vi "BRig_RT_panel_cue_v1,17.vi"(7 "input_setValues":bool, 11 "input_dataExp":u16[](array[numeric])) -> (3 "output_dataExp":u16[](array[numeric]))   [LabVIEW 2014]
panel:
  in  "Cue1B_LorR":bool
  in  "Cue1B_Prob":u16
  in  "sp__Cue1B":u16(slide)=2 max=2 step=1 scale=0.0..2.0
  in  "Audio_Amp__Cue1B":u16=100 caption="Amp"
  in  "Audio_Freq__Cue1B":u16=5 caption="Freq [kHz]" max=14 step=1
  in  "Cue1BSwitch_Prob":u16
  in  "Cue1BSwitch":u16(slide) max=3 step=1 scale=0.0..3.0
  in  "Cue2Switch_Count_PostR":u16
  in  "Cue2Switch_Prob_PostR":u16
  in  "Cue2Switch_PostR":u16(slide) max=3 step=1 scale=0.0..3.0
  in  "Cue2Switch_Count_PreR":u16
  in  "Cue2Switch_Count_First":u16
  in  "Cue2Switch_Prob_PreR":u16
  in  "Cue2Switch_PreR":u16(slide) max=3 step=1 scale=0.0..3.0
  in  "Cue2Switch_Prob_First":u16
  in  "Cue2Switch_First":u16(slide) max=3 step=1 scale=0.0..3.0
  in  "CueLed_baseline":bool
  in  "CueSwitch_Count_PostR":u16
  in  "CueSwitch_Prob_PostR":u16
  in  "CueSwitch_PostR":u16(slide) max=3 step=1 scale=0.0..3.0
  in  "CueSwitch_Count_PreR":u16
  in  "CueSwitch_Count_First":u16
  in  "CueSwitch_Prob_PreR":u16
  in  "CueSwitch_PreR":u16(slide) max=3 step=1 scale=0.0..3.0
  in  "CueSwitch_Prob_First":u16
  in  "CueSwitch_First":u16(slide) max=3 step=1 scale=0.0..3.0
  in  "CueLed_Freq":u16=10
  in  "CueLed_Tpeak":u16=2
  in  "sp_RightSpout":u16(slide)=2 max=2 step=1 scale=0.0..2.0
  in  "sp_LeftSpout":u16(slide)=2 max=2 step=1 scale=0.0..2.0
  in  "Audio_Amp__R":u16=100 caption="Amp"
  in  "Audio_Freq__R":u16=5 caption="Freq [kHz]" max=14 step=1
  in  "Audio_Amp__L":u16=100 caption="Amp"
  in  "Audio_Freq__L":u16=5 caption="Freq [kHz]" max=14 step=1
  # "Cue State\n                                             Cue Type         LED Probability    Count"
  # "Cue LED Parameters"
  # "Audio or LED"
  # "Frequency\n[Hz]"
  # "1A     1B"
  # "Timing [ms]\n                    Peak Width"
  # "1A\n1B"
  # "First"
  # "Pre Reward"
  # "Audio Parameters"
  # "Post Reward"
  # "Left                  Right"
  # "Frequency\n[kHz]"
  # "Cue2 State\n                                             Cue Type     LED Probability    Count"
  # "1A\n1B"
  # "2"
  # "Audio or LED"
  # "First"
  # "Amp\n(0 - 32,000)"
  # "1A\n1B"
  # "2"
  # "Pre Reward"
  # "1A  1B"
  # "2"
  # "Speaker\nPattern\nDuring Cue"
  # "Post Reward"
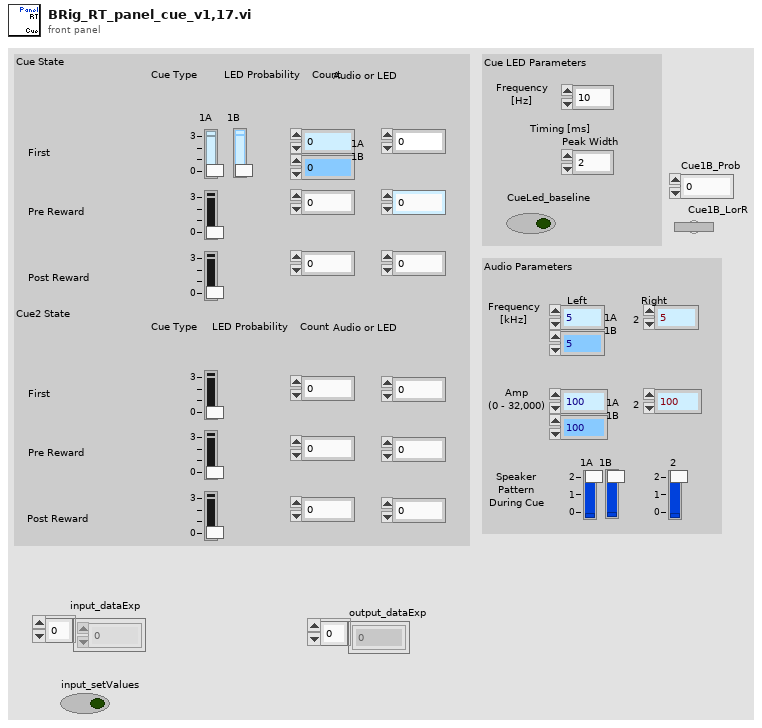
[diagram p1: front panel]
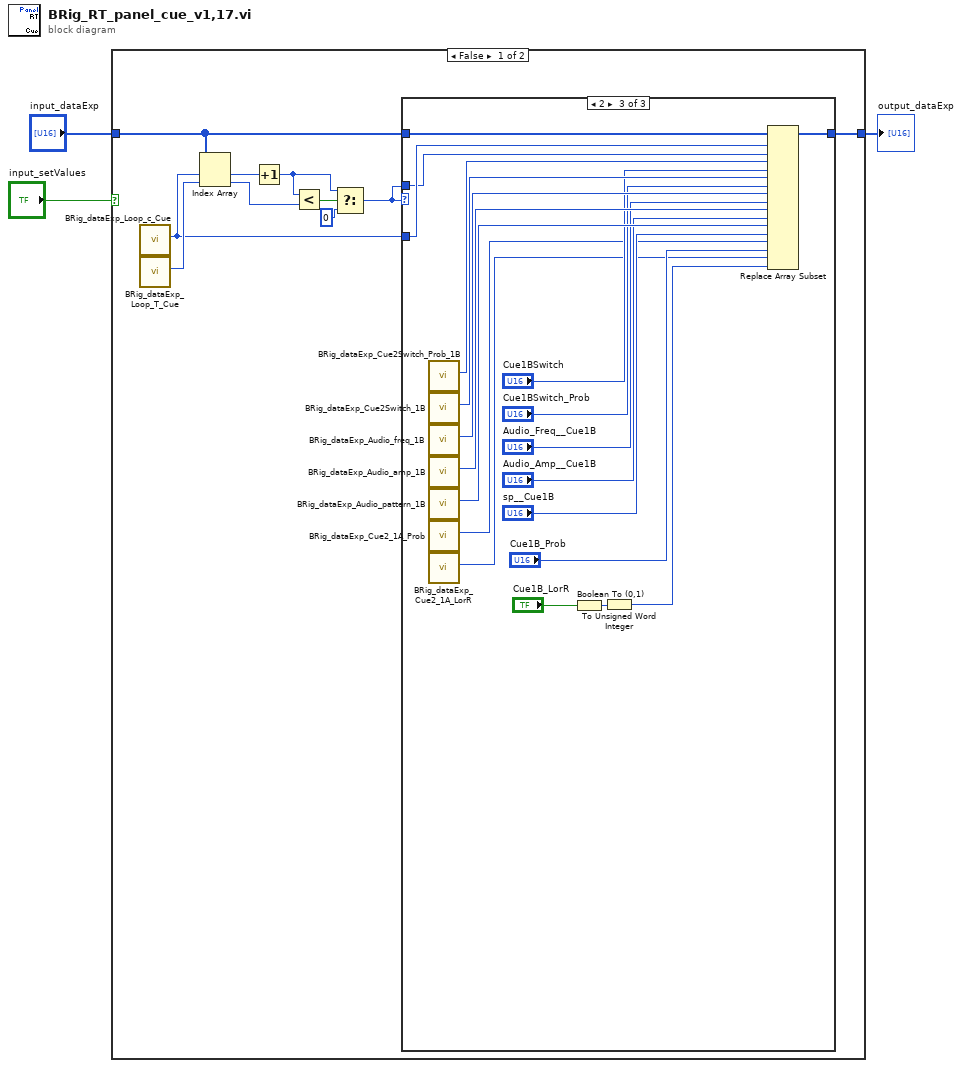
[diagram p0: block diagram]
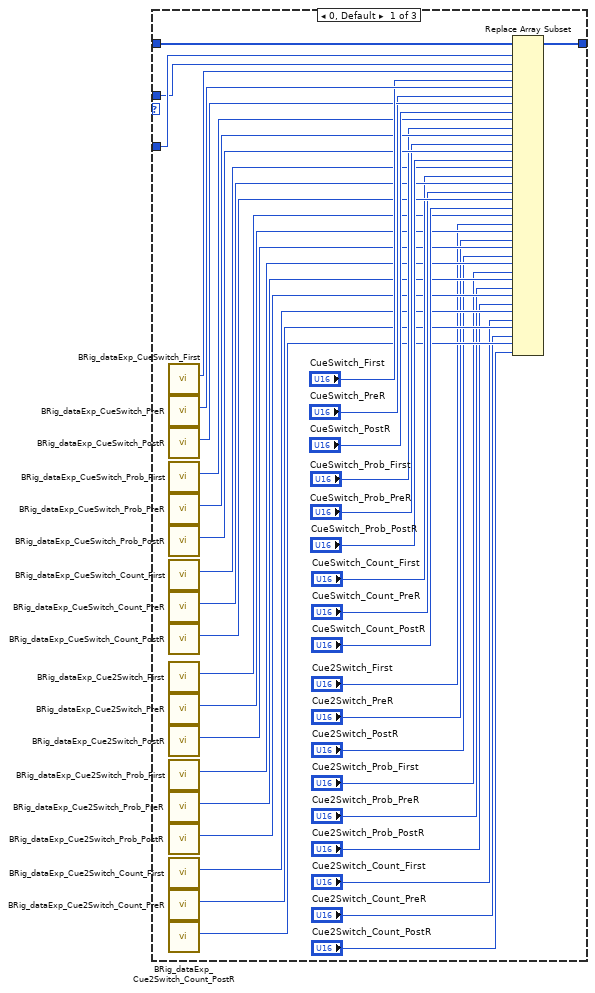
[diagram p2: hidden frame]
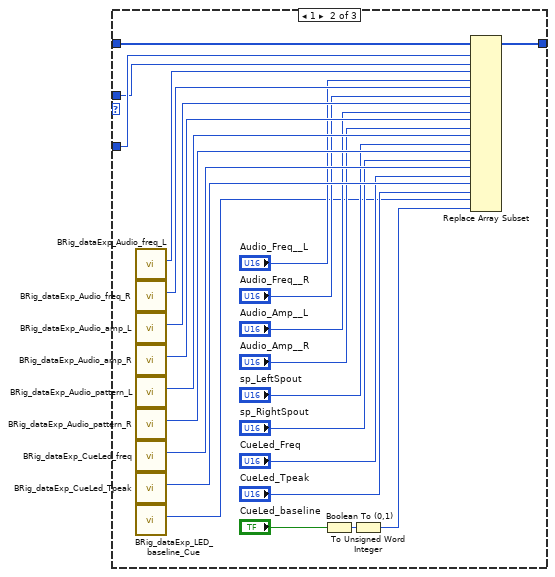
[diagram p3: hidden frame]
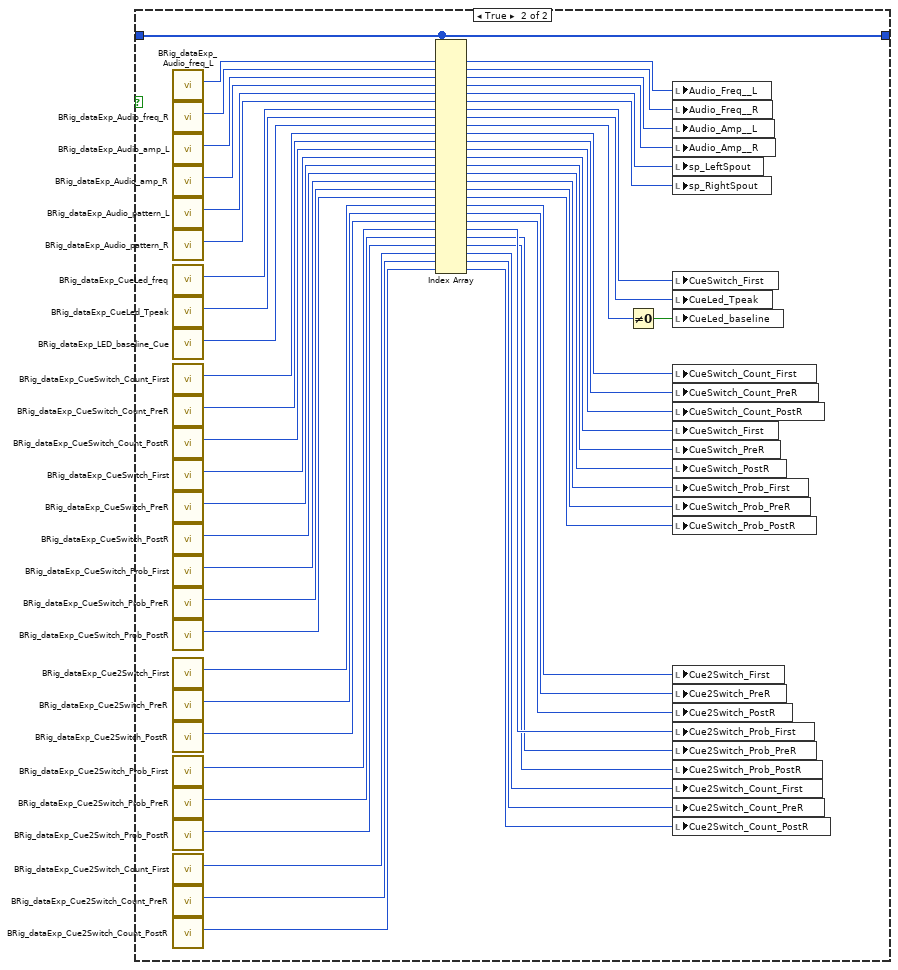
[diagram p4: hidden frame]
diagram:
  n1 = case shown="False" "input_setValues" {
    tunnel: "input_dataExp" -> [w7 w153]
    tunnel: [w6 w153] -> w2
    frame False {
      n2 = call "BRig_dataExp_Loop_c_Cue.vi"() -> ("output_Loop_c_Cue"=w5:i32)  [unwired: 11 in]
      n3 = call "BRig_dataExp_Loop_T_Cue.vi"() -> ("output_Loop_T_Cue"=w13:i32)  [unwired: 11 in]
      n4 = Index Array(array=w7, index #1=w5, index #2=w13) -> (element #1=w12:u16, element #2=w11:u16)
      n5 = Increment(x=w12) -> (x+1=w9:u16)
      n6 = Less?(x=w9, y=w11) -> (x < y?=w10:bool)
      n7 = Select(t=w9, s=w10, f=u16 0) -> (s? t:f=w4:u16)
      n8 = case shown="2" w4 {
        tunnel: w7 -> [w53 w77 w97]
        tunnel: [w34 w76 w96] -> w6
        tunnel: w5 -> [w33 w75 w95]
        tunnel: w4 -> [w32 w74 w94]
        frame 0, Default {
          n9 = call "BRig_dataExp_CueSwitch_First.vi"() -> ("output_CueSwitch_First"=w52:i32)  [unwired: 11 in]
          n10 = call "BRig_dataExp_CueSwitch_PreR.vi"() -> ("output_CueSwitch_PreR"=w51:i32)  [unwired: 11 in]
          n11 = call "BRig_dataExp_CueSwitch_PostR.vi"() -> ("output_CueSwitch_PostR"=w49:i32)  [unwired: 11 in]
          n12 = call "BRig_dataExp_CueSwitch_Prob_First.vi"() -> ("output_CueSwitch_Prob_First"=w46:i32)  [unwired: 11 in]
          n13 = call "BRig_dataExp_CueSwitch_Prob_PreR.vi"() -> ("output_CueSwitch_Prob_PreR"=w45:i32)  [unwired: 11 in]
          n14 = call "BRig_dataExp_CueSwitch_Prob_PostR.vi"() -> ("output_CueSwitch_Prob_PostR"=w44:i32)  [unwired: 11 in]
          n15 = call "BRig_dataExp_CueSwitch_Count_First.vi"() -> ("output_CueSwitch_Count_First"=w40:i32)  [unwired: 11 in]
          n16 = call "BRig_dataExp_CueSwitch_Count_PreR.vi"() -> ("output_CueSwitch_Count_PreR"=w39:i32)  [unwired: 11 in]
          n17 = call "BRig_dataExp_CueSwitch_Count_PostR.vi"() -> ("output_CueSwitch_Count_PostR"=w38:i32)  [unwired: 11 in]
          n18 = call "BRig_dataExp_Cue2Switch_First.vi"() -> ("output_Cue2Switch_First"=w31:i32)  [unwired: 11 in]
          n19 = call "BRig_dataExp_Cue2Switch_PreR.vi"() -> ("output_Cue2Switch_PreR"=w30:i32)  [unwired: 11 in]
          n20 = call "BRig_dataExp_Cue2Switch_PostR.vi"() -> ("output_Cue2Switch_PostR"=w29:i32)  [unwired: 11 in]
          n21 = call "BRig_dataExp_Cue2Switch_Prob_First.vi"() -> ("output_Cue2Switch_Prob_First"=w28:i32)  [unwired: 11 in]
          n22 = call "BRig_dataExp_Cue2Switch_Prob_PreR.vi"() -> ("output_Cue2Switch_Prob_PreR"=w27:i32)  [unwired: 11 in]
          n23 = call "BRig_dataExp_Cue2Switch_Prob_PostR.vi"() -> ("output_Cue2Switch_Prob_PostR"=w26:i32)  [unwired: 11 in]
          n24 = call "BRig_dataExp_Cue2Switch_Count_First.vi"() -> ("output_Cue2Switch_Count_First"=w25:i32)  [unwired: 11 in]
          n25 = call "BRig_dataExp_Cue2Switch_Count_PreR.vi"() -> ("output_Cue2Switch_Count_PreR"=w24:i32)  [unwired: 11 in]
          n26 = call "BRig_dataExp_Cue2Switch_Count_PostR.vi"() -> ("output_Cue2Switch_Count_PostR"=w23:i32)  [unwired: 11 in]
          n27 = Replace Array Subset(array=w53, new element #1=w32, index #1=w33, new element #2="CueSwitch_First", index #2=w52, new element #3="CueSwitch_PreR", index #3=w51, new element #4="CueSwitch_PostR", index #4=w49, new element #5="CueSwitch_Prob_First", index #5=w46, new element #6="CueSwitch_Prob_PreR", index #6=w45, new element #7="CueSwitch_Prob_PostR", index #7=w44, new element #8="CueSwitch_Count_First", index #8=w40, new element #9="CueSwitch_Count_PreR", index #9=w39, new element #10="CueSwitch_Count_PostR", index #10=w38, new element #11="Cue2Switch_First", index #11=w31, new element #12="Cue2Switch_PreR", index #12=w30, new element #13="Cue2Switch_PostR", index #13=w29, new element #14="Cue2Switch_Prob_First", index #14=w28, new element #15="Cue2Switch_Prob_PreR", index #15=w27, new element #16="Cue2Switch_Prob_PostR", index #16=w26, new element #17="Cue2Switch_Count_First", index #17=w25, new element #18="Cue2Switch_Count_PreR", index #18=w24, new element #19="Cue2Switch_Count_PostR", index #19=w23) -> (w34:u16[])
        }
        frame 1 {
          n28 = call "BRig_dataExp_Audio_freq_L.vi"() -> ("output_Audio_freq__L"=w73:i32)  [unwired: 11 in]
          n29 = call "BRig_dataExp_Audio_freq_R.vi"() -> ("output_Audio_freq__R"=w72:i32)  [unwired: 11 in]
          n30 = call "BRig_dataExp_Audio_amp_L.vi"() -> ("output_Audio_amp__L"=w71:i32)  [unwired: 11 in]
          n31 = call "BRig_dataExp_Audio_amp_R.vi"() -> ("output_Audio_amp__R"=w70:i32)  [unwired: 11 in]
          n32 = call "BRig_dataExp_Audio_pattern_L.vi"() -> ("output_Audio_sp__L"=w69:i32)  [unwired: 11 in]
          n33 = call "BRig_dataExp_Audio_pattern_R.vi"() -> ("output_Audio_sp__R"=w68:i32)  [unwired: 11 in]
          n34 = call "BRig_dataExp_CueLed_freq.vi"() -> ("output_CueLed_Freq"=w67:i32)  [unwired: 11 in]
          n35 = call "BRig_dataExp_CueLed_Tpeak.vi"() -> ("output_CueLed_Tpeak"=w66:i32)  [unwired: 11 in]
          n36 = call "BRig_dataExp_LED_baseline_Cue.vi"() -> ("output_LED_baseline_Cue"=w57:i32)  [unwired: 11 in]
          n37 = Boolean To (0,1)(Boolean="CueLed_baseline") -> (0, 1=w55:i16)
          n38 = To Unsigned Word Integer(number=w55) -> (unsigned 16bit integer=w54:u16)
          n39 = Replace Array Subset(array=w77, new element #1=w74, index #1=w75, new element #2="Audio_Freq__L", index #2=w73, new element #3="Audio_Freq__R", index #3=w72, new element #4="Audio_Amp__L", index #4=w71, new element #5="Audio_Amp__R", index #5=w70, new element #6="sp_LeftSpout", index #6=w69, new element #7="sp_RightSpout", index #7=w68, new element #8="CueLed_Freq", index #8=w67, new element #9="CueLed_Tpeak", index #9=w66, new element #10=w54, index #10=w57) -> (w76:u16[])
        }
        frame 2 {
          n40 = call "BRig_dataExp_Cue2Switch_Prob_1B.vi"() -> ("output_Cue2Switch_Prob_1B"=w93:i32)  [unwired: 11 in]
          n41 = call "BRig_dataExp_Cue2Switch_1B.vi"() -> ("output_Cue2Switch_1B"=w92:i32)  [unwired: 11 in]
          n42 = call "BRig_dataExp_Audio_freq_1B.vi"() -> ("output_Audio_freq__1B"=w91:i32)  [unwired: 11 in]
          n43 = call "BRig_dataExp_Audio_amp_1B.vi"() -> ("output_Audio_amp__1B"=w90:i32)  [unwired: 11 in]
          n44 = call "BRig_dataExp_Audio_pattern_1B.vi"() -> ("output_Audio_sp__1B"=w89:i32)  [unwired: 11 in]
          n45 = call "BRig_dataExp_Cue2_1A_Prob.vi"() -> ("output_Cue2_1A_Prob"=w83:i32)  [unwired: 11 in]
          n46 = call "BRig_dataExp_Cue2_1A_LorR.vi"() -> ("output_Cue2_1A_LorR"=w81:i32)  [unwired: 11 in]
          n47 = Boolean To (0,1)(Boolean="Cue1B_LorR") -> (0, 1=w79:i16)
          n48 = To Unsigned Word Integer(number=w79) -> (unsigned 16bit integer=w78:u16)
          n49 = Replace Array Subset(array=w97, new element #1=w94, index #1=w95, new element #2="Cue1BSwitch", index #2=w93, new element #3="Cue1BSwitch_Prob", index #3=w92, new element #4="Audio_Freq__Cue1B", index #4=w91, new element #5="Audio_Amp__Cue1B", index #5=w90, new element #6="sp__Cue1B", index #6=w89, new element #7="Cue1B_Prob", index #7=w83, new element #8=w78, index #8=w81) -> (w96:u16[])
        }
      }
    }
    frame True {
      n50 = call "BRig_dataExp_Audio_freq_L.vi"() -> ("output_Audio_freq__L"=w152:i32)  [unwired: 11 in]
      n51 = call "BRig_dataExp_Audio_freq_R.vi"() -> ("output_Audio_freq__R"=w150:i32)  [unwired: 11 in]
      n52 = call "BRig_dataExp_Audio_amp_L.vi"() -> ("output_Audio_amp__L"=w148:i32)  [unwired: 11 in]
      n53 = call "BRig_dataExp_Audio_amp_R.vi"() -> ("output_Audio_amp__R"=w146:i32)  [unwired: 11 in]
      n54 = call "BRig_dataExp_Audio_pattern_L.vi"() -> ("output_Audio_sp__L"=w144:i32)  [unwired: 11 in]
      n55 = call "BRig_dataExp_Audio_pattern_R.vi"() -> ("output_Audio_sp__R"=w143:i32)  [unwired: 11 in]
      n56 = call "BRig_dataExp_CueLed_freq.vi"() -> ("output_CueLed_Freq"=w140:i32)  [unwired: 11 in]
      n57 = call "BRig_dataExp_CueLed_Tpeak.vi"() -> ("output_CueLed_Tpeak"=w138:i32)  [unwired: 11 in]
      n58 = call "BRig_dataExp_LED_baseline_Cue.vi"() -> ("output_LED_baseline_Cue"=w136:i32)  [unwired: 11 in]
      n59 = call "BRig_dataExp_CueSwitch_Count_First.vi"() -> ("output_CueSwitch_Count_First"=w133:i32)  [unwired: 11 in]
      n60 = call "BRig_dataExp_CueSwitch_Count_PreR.vi"() -> ("output_CueSwitch_Count_PreR"=w132:i32)  [unwired: 11 in]
      n61 = call "BRig_dataExp_CueSwitch_Count_PostR.vi"() -> ("output_CueSwitch_Count_PostR"=w131:i32)  [unwired: 11 in]
      n62 = call "BRig_dataExp_CueSwitch_First.vi"() -> ("output_CueSwitch_First"=w130:i32)  [unwired: 11 in]
      n63 = call "BRig_dataExp_CueSwitch_PreR.vi"() -> ("output_CueSwitch_PreR"=w129:i32)  [unwired: 11 in]
      n64 = call "BRig_dataExp_CueSwitch_PostR.vi"() -> ("output_CueSwitch_PostR"=w128:i32)  [unwired: 11 in]
      n65 = call "BRig_dataExp_CueSwitch_Prob_First.vi"() -> ("output_CueSwitch_Prob_First"=w127:i32)  [unwired: 11 in]
      n66 = call "BRig_dataExp_CueSwitch_Prob_PreR.vi"() -> ("output_CueSwitch_Prob_PreR"=w126:i32)  [unwired: 11 in]
      n67 = call "BRig_dataExp_CueSwitch_Prob_PostR.vi"() -> ("output_CueSwitch_Prob_PostR"=w125:i32)  [unwired: 11 in]
      n68 = call "BRig_dataExp_Cue2Switch_First.vi"() -> ("output_Cue2Switch_First"=w115:i32)  [unwired: 11 in]
      n69 = call "BRig_dataExp_Cue2Switch_PreR.vi"() -> ("output_Cue2Switch_PreR"=w114:i32)  [unwired: 11 in]
      n70 = call "BRig_dataExp_Cue2Switch_PostR.vi"() -> ("output_Cue2Switch_PostR"=w113:i32)  [unwired: 11 in]
      n71 = call "BRig_dataExp_Cue2Switch_Prob_First.vi"() -> ("output_Cue2Switch_Prob_First"=w112:i32)  [unwired: 11 in]
      n72 = call "BRig_dataExp_Cue2Switch_Prob_PreR.vi"() -> ("output_Cue2Switch_Prob_PreR"=w111:i32)  [unwired: 11 in]
      n73 = call "BRig_dataExp_Cue2Switch_Prob_PostR.vi"() -> ("output_Cue2Switch_Prob_PostR"=w110:i32)  [unwired: 11 in]
      n74 = call "BRig_dataExp_Cue2Switch_Count_First.vi"() -> ("output_Cue2Switch_Count_First"=w109:i32)  [unwired: 11 in]
      n75 = call "BRig_dataExp_Cue2Switch_Count_PreR.vi"() -> ("output_Cue2Switch_Count_PreR"=w108:i32)  [unwired: 11 in]
      n76 = call "BRig_dataExp_Cue2Switch_Count_PostR.vi"() -> ("output_Cue2Switch_Count_PostR"=w107:i32)  [unwired: 11 in]
      n77 = Index Array(array=w153, index #1=w152, index #2=w150, index #3=w148, index #4=w146, index #5=w144, index #6=w143, index #7=w140, index #8=w138, index #9=w136, index #10=w133, index #11=w132, index #12=w131, index #13=w130, index #14=w129, index #15=w128, index #16=w127, index #17=w126, index #18=w125, index #19=w115, index #20=w114, index #21=w113, index #22=w112, index #23=w111, index #24=w110, index #25=w109, index #26=w108, index #27=w107) -> (element #1=w151:u16, element #2=w149:u16, element #3=w147:u16, element #4=w145:u16, element #5=w142:u16, element #6=w141:u16, element #7=w139:u16, element #8=w137:u16, element #9=w134:u16, element #10=w124:u16, element #11=w123:u16, element #12=w122:u16, element #13=w121:u16, element #14=w120:u16, element #15=w119:u16, element #16=w118:u16, element #17=w117:u16, element #18=w116:u16, element #19=w106:u16, element #20=w105:u16, element #21=w104:u16, element #22=w103:u16, element #23=w102:u16, element #24=w101:u16, element #25=w100:u16, element #26=w99:u16, element #27=w98:u16)
      n78 = Not Equal To 0?(x=w134) -> (x != 0?=w135:bool)
      n79 = local write "Audio_Freq__L"(w151) -> ()
      n80 = local write "Audio_Freq__R"(w149) -> ()
      n81 = local write "Audio_Amp__L"(w147) -> ()
      n82 = local write "Audio_Amp__R"(w145) -> ()
      n83 = local write "sp_LeftSpout"(w142) -> ()
      n84 = local write "sp_RightSpout"(w141) -> ()
      n85 = local write "CueSwitch_First"(w139) -> ()
      n86 = local write "CueLed_Tpeak"(w137) -> ()
      n87 = local write "CueLed_baseline"(w135) -> ()
      n88 = local write "CueSwitch_Count_First"(w124) -> ()
      n89 = local write "CueSwitch_Count_PreR"(w123) -> ()
      n90 = local write "CueSwitch_Count_PostR"(w122) -> ()
      n91 = local write "CueSwitch_First"(w121) -> ()
      n92 = local write "CueSwitch_PreR"(w120) -> ()
      n93 = local write "CueSwitch_PostR"(w119) -> ()
      n94 = local write "CueSwitch_Prob_First"(w118) -> ()
      n95 = local write "CueSwitch_Prob_PreR"(w117) -> ()
      n96 = local write "CueSwitch_Prob_PostR"(w116) -> ()
      n97 = local write "Cue2Switch_First"(w106) -> ()
      n98 = local write "Cue2Switch_PreR"(w105) -> ()
      n99 = local write "Cue2Switch_PostR"(w104) -> ()
      n100 = local write "Cue2Switch_Prob_First"(w103) -> ()
      n101 = local write "Cue2Switch_Prob_PreR"(w102) -> ()
      n102 = local write "Cue2Switch_Prob_PostR"(w101) -> ()
      n103 = local write "Cue2Switch_Count_First"(w100) -> ()
      n104 = local write "Cue2Switch_Count_PreR"(w99) -> ()
      n105 = local write "Cue2Switch_Count_PostR"(w98) -> ()
    }
  }
  "output_dataExp" <- w2
